vi "Main.CheckAddressClaim.vi"(8 "error in (no error)":errorcluster, 11 "Protocol App":T1={"XNET Settings"={"Database"="", "Cluster"="", "Port"="", "Baud rate [Bd]"=0, "Termination"=0, "Incoming Rate"=0, "Outcoming Rate"=1, "Write Decimation"=1}, "Data"=[], "DTCs"=[], "Sim Addresses LUT"=variant, "Data Table LUT"=variant, "MonitorTool.Network"={"Address"=0, "Name"=0}, "Name"=""} {"MonitorTool.Network"."Name" format="%.0x"; "DTCs"."Data"."DM1 Ref"."Data Reference" format="%.0x"; "DTCs"."Data"."DM1 Enable Ref"."Data Reference" format="%.0x"; "DTCs"."Data"."DM2 Ref"."Data Reference" format="%.0x"; "DTCs"."Data"."DM2 Enable Ref"."Data Reference" format="%.0x"; "Data"."Network"."Name" format="%.0x"; "Data"."IncomingRefs"."Data Reference" format="%.0x"; "Data"."OutgoingRefs"."Data Reference" format="%.0x"; "XNET Settings"."Termination" items=["Off", "On"]}) -> (0 "error out":errorcluster, 3 "Address Claim Error":bool)   [LabVIEW 2015, in "J1939 Addon Engine.lvlib"]
uses:
  J1939 Addon Engine.lvlib
  Types/Protocol.App Settings.ctl
  Shared/Types/XNET Settings.ctl
  Types/Protocol.XNET Refs.ctl
  <vilib>/NI Veristand/Custom Device API/Block Data Reference.ctl
  <vilib>/NI Veristand/Custom Device API/Data Reference.ctl
  Shared/Types/Monitor Settings.ctl
  Types/Engine.DTC Settings.ctl
  Shared/Types/Compiled Simulated Settings.ctl
  Types/Engine.DTC FIFOs.ctl
  <vilib>/xnet/xnet.llb/XNET Read (State J1939 Comm).vi
  Shared/J1939 Addon Shared.lvlib
  <vilib>/NI VeriStand/Custom Device API/Custom Device API.lvlib
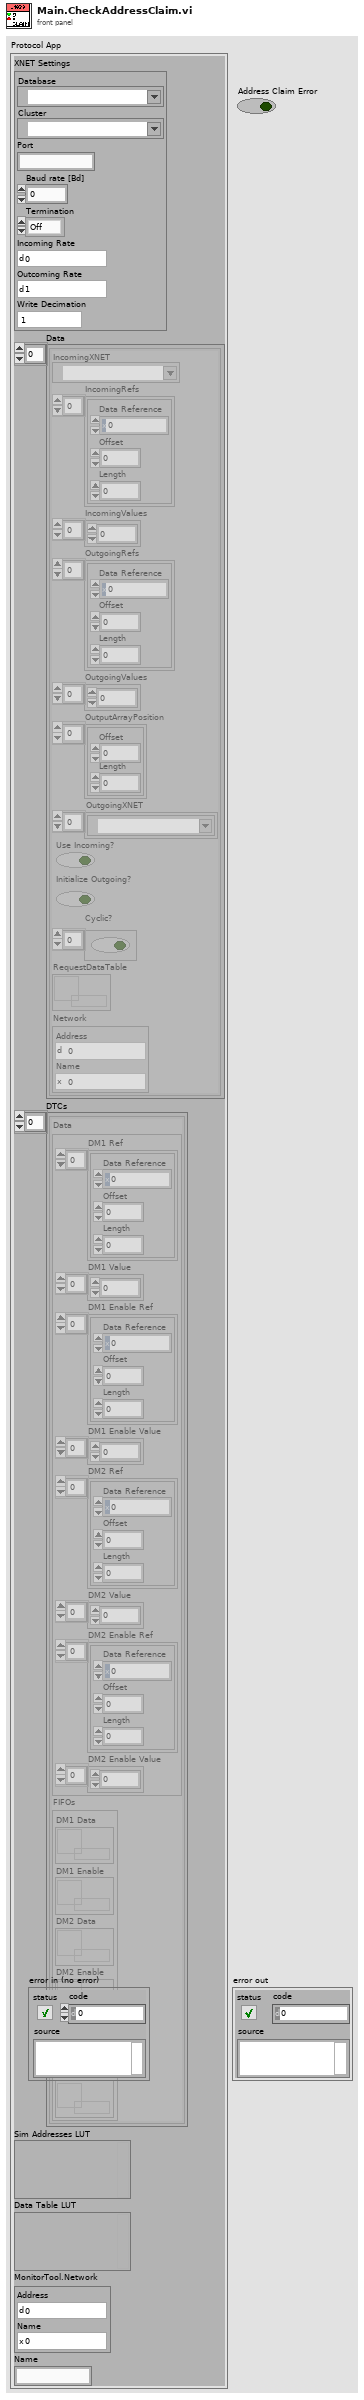
[diagram p1: front panel]
types:
  T1 = typedef "J1939 Addon Engine.lvlib/Protocol.App Settings.ctl" = cluster{"XNET Settings":T2, "Data":T3[], "DTCs":T7[], "Sim Addresses LUT":variant, "Data Table LUT":variant, "MonitorTool.Network":T6, "Name":string}
  T2 = typedef "J1939 Addon Shared.lvlib/XNET Settings.ctl" = cluster{"Database":refnum<k21>, "Cluster":refnum<k21>, "Port":string, "Baud rate [Bd]":u32, "Termination":u32, "Incoming Rate":u32, "Outcoming Rate":u32, "Write Decimation":u32}
  T3 = typedef "J1939 Addon Engine.lvlib/Protocol.XNET Refs.ctl" = cluster{"IncomingXNET":refnum<k21>, "IncomingRefs":T4[], "IncomingValues":dbl[], "OutgoingRefs":T4[], "OutgoingValues":dbl[], "OutputArrayPosition":cluster{"Offset":u32, "Length":u32}[], "OutgoingXNET":refnum<k21>[], "Use Incoming?":bool, "Initialize Outgoing?":bool, "Cyclic?":bool[], "RequestDataTable":refnum<k33>, "Network":T6}
  T4 = typedef "Custom Device API.lvlib/Block Data Reference.ctl" = cluster{"Data Reference":T5, "Offset":u64, "Length":u64}
  T5 = typedef "Custom Device API.lvlib/Data Reference.ctl" = i32
  T6 = typedef "J1939 Addon Shared.lvlib/Monitor Settings.ctl" = cluster{"Address":u8, "Name":u64}
  T7 = typedef "J1939 Addon Engine.lvlib/Engine.DTC Settings.ctl" = cluster{"Data":T8, "FIFOs":T9}
  T8 = typedef "J1939 Addon Shared.lvlib/Compiled Simulated Settings.ctl" = cluster{"DM1 Ref":T4[], "DM1 Value":dbl[], "DM1 Enable Ref":T4[], "DM1 Enable Value":dbl[], "DM2 Ref":T4[], "DM2 Value":dbl[], "DM2 Enable Ref":T4[], "DM2 Enable Value":dbl[]}
  T9 = typedef "J1939 Addon Engine.lvlib/Engine.DTC FIFOs.ctl" = cluster{"DM1 Data":refnum<k33>, "DM1 Enable":refnum<k33>, "DM2 Data":refnum<k33>, "DM2 Enable":refnum<k33>, "DM1 Reset":refnum<k33>, "DM2 Reset":refnum<k33>}
  T10 = typedef "XNET J1939 Comm.ctl" = cluster{"fault code":i32, "fault?":bool, "PGN":u32, "src addr":u8, "dest addr":u8, "transmit error":bool, "receive error":bool}
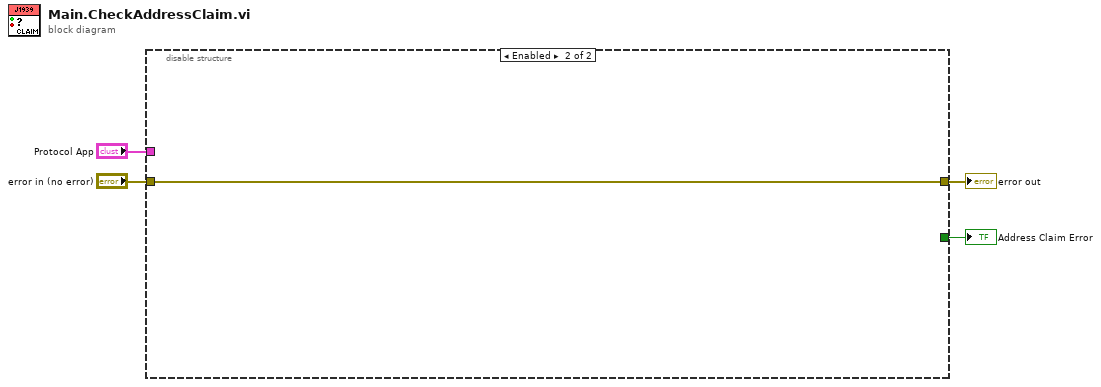
[diagram p0: block diagram]
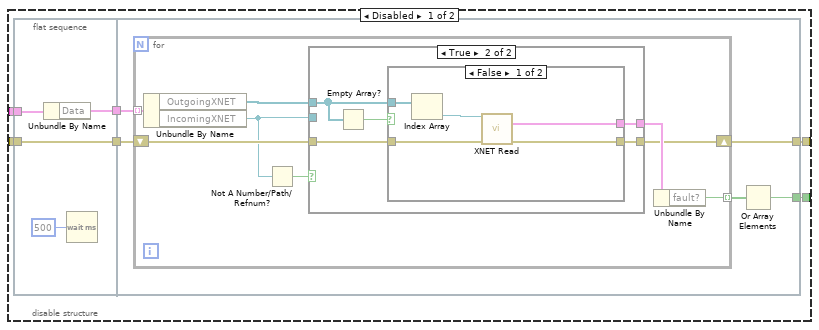
[diagram p2: hidden frame]
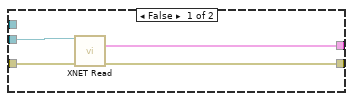
[diagram p3: hidden frame]
diagram:
  n1 = disable-structure shown="Enabled" {
    disable-tunnel: [w8 _] -> w4
    disable-tunnel: [w7 w43] -> w3
    disable-tunnel: "Protocol App" -> [w6 _]
    disable-tunnel: "error in (no error)" -> [w5 w43]
    frame Disabled {
      n2 = flat-sequence {
        tunnel: [w11] -> w10
        tunnel: [w13] -> w9
        tunnel: w5 -> [w13]
        tunnel: w6 -> [w12]
        tunnel: w10 -> [w19]
        tunnel: w9 -> [w18]
        tunnel: [w16] -> w8
        tunnel: [w15] -> w7
        frame #0 {
          n3 = Unbundle By Name(w12) -> ("Data"=w11:T3[])
          n4 = Wait (ms)(milliseconds to wait=u32 500) -> ()  [unwired: 1 out]
        }
        frame #1 {
          n5 = for {
            tunnel: w19 -> [w27] mode=indexing
            shift-right: [w20] -> w15
            shift-left: w18 -> [w26]
            tunnel: [w21] -> w17 mode=indexing
            n6 = Unbundle By Name(w27) -> ("OutgoingXNET"=w22:refnum<k21>[], "IncomingXNET"=w24:refnum<k21>)
            n7 = Not A Number/Path/Refnum?(number/path/refnum=w24) -> (NaN/Path/Refnum?=w23:bool)
            n8 = case shown="True" w23 {
              tunnel: w26 -> [w31 w34]
              tunnel: [w30 w33] -> w25
              tunnel: [w29 w32] -> w20
              tunnel: w24 -> [w28 _]
              tunnel: w22 -> [_ w35]
              frame False {
                n9 = call-poly <vilib>:"XNET Read.vi"("session in"=w28, "error in (no error)"=w31) -> ("J1939 comm"=w30:T10, "error out"=w29:errorcluster)  [unwired: 11 in, 1 out]
              }
              frame True {
                n10 = Empty Array?(array=w35) -> (empty?=w36:bool)
                n11 = case shown="False" w36 {
                  tunnel: w35 -> [w41 _]
                  tunnel: w34 -> [w39 w42]
                  tunnel: [w38 _] -> w33
                  tunnel: [w37 w42] -> w32
                  frame False {
                    n12 = Index Array(array=w41) -> (element=w40:refnum<k21>)  [unwired: 1 in]
                    n13 = call-poly <vilib>:"XNET Read.vi"("session in"=w40, "error in (no error)"=w39) -> ("J1939 comm"=w38:T10, "error out"=w37:errorcluster)  [unwired: 11 in, 1 out]
                  }
                  frame True {
                  }
                }
              }
            }
            n14 = Unbundle By Name(w25) -> ("fault?"=w21:bool)
          }
          n15 = Or Array Elements(Boolean array=w17) -> (logical OR=w16:bool)
        }
      }
    }
    frame Enabled {
    }
  }
  "Address Claim Error" <- w4
  "error out" <- w3
